vi "Review Branch.vi"(8 "error in":errorcluster, 11 "Peer Review in":refnum<class "Peer Review.lvclass">) -> (0 "error out":errorcluster, 3 "Peer Review out":refnum<class "Peer Review.lvclass">)   [LabVIEW 2020, in "Peer Review.lvclass"]
uses:
  Peer Review.lvclass
  Peer Review.lvclass/Peer Review.ctl
  <vilib>/Utility/cursorutil.llb/Set Cursor (Icon Pict).vi
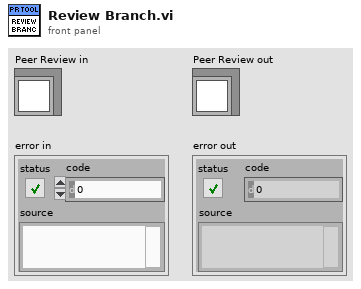
[diagram p1: front panel]
types:
  T1 = enum32{"Commit History", "File List", "Git Log", "Description", "Image"}
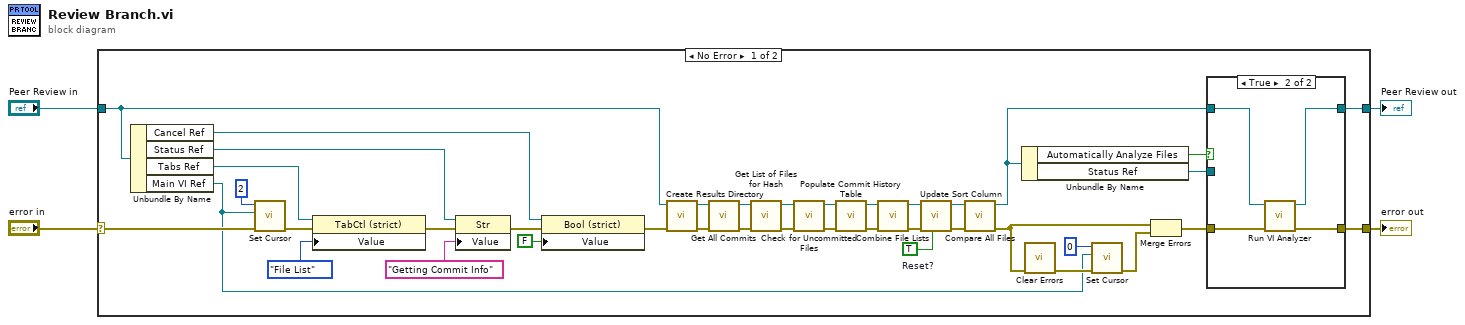
[diagram p0: block diagram]
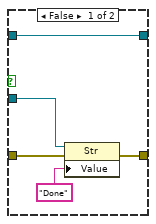
[diagram p2: hidden frame]
diagram:
  n1 = case shown="No Error" "error in" {
    selector: "error in" -> [w20 w54]
    tunnel: [w31 w54] -> w4
    tunnel: "Peer Review in" -> [w17 w53]
    tunnel: [w33 w53] -> w1
    frame No Error {
      w32 = TRUE  # Reset?
      n2 = Unbundle By Name(w17) -> ("Cancel Ref"=w7:refnum<vi>, "Status Ref"=w35:refnum<vi>, "Tabs Ref"=w37:refnum<vi>, "Main VI Ref"=w12:refnum<vi>)
      n3 = call-poly <vilib>:"Set Cursor.vi"("error in (no error)"=w20, "VI reference (current VI)"=w12, "icon"=u16 2) -> ("error out"=w19:errorcluster)  [unwired: 7 in, 1 out]
      n4 = property on="Property Node" class="TabCtl (strict)"(reference=w37, error in=w19, "Value"=T1."File List") -> (error out=w36:errorcluster)  [unwired: 1 out]
      n5 = property on="Property Node" class="Str"(reference=w35, error in=w36, "Value"="Getting Commit Info") -> (error out=w8:errorcluster)  [unwired: 1 out]
      n6 = property on="Property Node" class="Bool (strict)"(reference=w7, error in=w8, "Value"=FALSE) -> (error out=w5:errorcluster)  [unwired: 1 out]
      n7 = call "Create Results Directory.vi"("error in"=w5, "Peer Review in"=w17) -> ("error out"=w43:errorcluster, "Peer Review out"=w40:refnum<class "Peer Review.lvclass">)  [unwired: 8 in]
      n8 = call "Get All Commits.vi"("error in"=w43, "Peer Review in"=w40) -> ("error out"=w39:errorcluster, "Peer Review out"=w38:refnum<class "Peer Review.lvclass">)  [unwired: 8 in]
      n9 = call "Get List of Files for Hash.vi"("error in"=w39, "Peer Review in"=w38) -> ("error out"=w26:errorcluster, "Peer Review out"=w27:refnum<class "Peer Review.lvclass">)  [unwired: 8 in]
      n10 = call "Check for Uncommitted Files.vi"("error in"=w26, "Peer Review in"=w27) -> ("error out"=w25:errorcluster, "Peer Review out"=w24:refnum<class "Peer Review.lvclass">)  [unwired: 8 in]
      n11 = call "Populate Commit History Table.vi"("error in"=w25, "Peer Review in"=w24) -> ("error out"=w29:errorcluster, "Peer Review out"=w28:refnum<class "Peer Review.lvclass">)  [unwired: 8 in]
      n12 = call "Combine File Lists.vi"("error in"=w29, "Peer Review in"=w28) -> ("error out"=w41:errorcluster, "Peer Review out"=w42:refnum<class "Peer Review.lvclass">)  [unwired: 8 in]
      n13 = call "Update Sort Column.vi"("Reset?"=w32, "error in"=w41, "Peer Review in"=w42) -> ("error out"=w22:errorcluster, "Peer Review out"=w23:refnum<class "Peer Review.lvclass">)  [unwired: 7 in]
      n14 = call "Compare All Files.vi"("error in"=w22, "Peer Review in"=w23) -> ("error out"=w10:errorcluster, "Peer Review out"=w15:refnum<class "Peer Review.lvclass">)  [unwired: 8 in]
      n15 = Unbundle By Name(w15) -> ("Automatically Analyze Files"=w16:bool, "Status Ref"=w14:refnum<vi>)
      n16 = call <vilib>:"Clear Errors.vi"("error in (no error)"=w10) -> ("error out"=w13:errorcluster)  [unwired: 5 in, 1 out]
      n17 = call-poly <vilib>:"Set Cursor.vi"("error in (no error)"=w13, "VI reference (current VI)"=w12, "icon"=u16 0) -> ("error out"=w11:errorcluster)  [unwired: 7 in, 1 out]
      n18 = Merge Errors(w10, w11) -> (w9:errorcluster)
      n19 = case shown="True" w16 {
        tunnel: w15 -> [w45 w52]
        tunnel: [w45 w51] -> w33
        tunnel: w9 -> [w47 w50]
        tunnel: [w46 w49] -> w31
        tunnel: w14 -> [w44 _]
        frame False {
          n20 = property on="Property Node" class="Str"(reference=w44, error in=w47, "Value"="Done") -> (error out=w46:errorcluster)  [unwired: 1 out]
        }
        frame True {
          n21 = call "Run VI Analyzer.vi"("error in"=w50, "Peer Review in"=w52) -> ("error out"=w49:errorcluster, "Peer Review out"=w51:refnum<class "Peer Review.lvclass">)  [unwired: 8 in]
        }
      }
    }
    frame Error {
    }
  }
  "error out" <- w4
  "Peer Review out" <- w1
